vi "nanocal -- nuclear schottky fit V8.vi"() -> ()   [LabVIEW 2021] (continued)
,  \"τN\" -> 0.000008203122   ,  \"τC\" -> 0.002636418134   ,  \"κ0\" -> 0.000000022540   ,  \"mm1\" -> 0.000036639898   ,  \"mm2\" -> 0.012730445827   ,  \"mm3\" -> 0.021569578789   ,  \"T\" -> 3.100000000000   ,  \"B\" -> 10.000000000000   ,  \"θ\" -> 90.000000000000   ,  \"Reoff\" -> -204081.632653061300   ,  \"Imoff\" -> 0.000000000000   ,  \"στ1\" -> 0.714525927996   ,  \"στS\" -> 0.000197909015   ,  \"στN\" -> 0.366603423191   ,  \"τ11 \" -> 0.000000000000   ,  \"τ12\" -> 0.000000000000   ,  \"τ22\" -> 0.000000000000   ,  \"τN1\" -> 0.000000000000   ,  \"τN2\" -> 0.000000000000   ,  \"σηlogτ1 \" -> 0.000000000000   ,  \"σηlogτS\" -> 0.000000000000   ,  \"σηlogτN\" -> 0.000000000000   ,  \"σlogτ1\" -> 0.000000000000   ,  \"σlogτS\" -> 0.000000000000   ,  \"σlogτN\" -> 0.000000000000   ,  \"σητ1\" -> 0.000000000000   ,  \"σητS \" -> 0.000000000000   ,  \"σητN\" -> 0.000000000000    |>   , \n\"IDS0637_220612_RAW_cal__sam_\" ->   <|    \"ζ\" -> 0.000000000000   ,  \"τ1\" -> 0.000000000000   ,  \"τS\" -> 0.000000000000   ,  \"τN\" -> 0.000000000000   ,  \"τC\" -> 0.000000000000   ,  \"κ0\" -> 0.000000000000   ,  \"mm1\" -> 0.000000000000   ,  \"mm2\" -> 0.000000000000   ,  \"mm3\" -> 0.000000000000   ,  \"T\" -> 3.100000000000   ,  \"B\" -> 10.000000000000   ,  \"θ\" -> 90.000000000000   ,  \"Reoff\" -> 0.000000000000   ,  \"Imoff\" -> 0.000000000000   ,  \"στ1\" -> 0.000000000000   ,  \"στS\" -> 0.000000000000   ,  \"στN\" -> 0.000000000000   ,  \"τ11 \" -> 0.000000000000   ,  \"τ12\" -> 0.000000000000   ,  \"τ22\" -> 0.000000000000   ,  \"τN1\" -> 0.000000000000   ,  \"τN2\" -> 0.000000000000   ,  \"σηlogτ1 \" -> 0.000000000000   ,  \"σηlogτS\" -> 0.000000000000   ,  \"σηlogτN\" -> 0.000000000000   ,  \"σlogτ1\" -> 0.000000000000   ,  \"σlogτS\" -> 0.000000000000   ,  \"σlogτN\" -> 0.000000000000   ,  \"σητ1\" -> 0.000000000000   ,  \"σητS \" -> 0.000000000000   ,  \"σητN\" -> 0.000000000000    |>   , \n\"IDS0638_220612_RAW_cal__ref_\" ->   <|    \"ζ\" -> 0.021698598791   ,  \"τ1\" -> 0.021496688345   ,  \"τS\" -> 0.006445256992   ,  \"τN\" -> 0.000001238561   ,  \"τC\" -> 0.001823286983   ,  \"κ0\" -> 0.000000055353   ,  \"mm1\" -> 0.000030436072   ,  \"mm2\" -> 0.008377153736   ,  \"mm3\" -> 0.021498760993   ,  \"T\" -> 5.700000000000   ,  \"B\" -> 10.000000000000   ,  \"θ\" -> 90.000000000000   ,  \"Reoff\" -> -122448.979591835290   ,  \"Imoff\" -> 0.000000000000   ,  \"στ1\" -> 9.353728365028   ,  \"στS\" -> 0.000421905194   ,  \"στN\" -> 5.932285308296   ,  \"τ11 \" -> 0.000000000000   ,  \"τ12\" -> 0.000000000000   ,  \"τ22\" -> 0.000000000000   ,  \"τN1\" -> 0.000000000000   ,  \"τN2\" -> 0.000000000000   ,  \"σηlogτ1 \" -> 0.000000000000   ,  \"σηlogτS\" -> 0.000000000000   ,  \"σηlogτN\" -> 0.000000000000   ,  \"σlogτ1\" -> 0.000000000000   ,  \"σlogτS\" -> 0.000000000000   ,  \"σlogτN\" -> 0.000000000000   ,  \"σητ1\" -> 0.000000000000   ,  \"σητS \" -> 0.000000000000   ,  \"σητN\" -> 0.000000000000    |>   , \n\"IDS0638_220612_RAW_cal__sam_\" ->   <|    \"ζ\" -> 0.000000000000   ,  \"τ1\" -> 0.000000000000   ,  \"τS\" -> 0.000000000000   ,  \"τN\" -> 0.000000000000   ,  \"τC\" -> 0.000000000000   ,  \"κ0\" -> 0.000000000000   ,  \"mm1\" -> 0.000000000000   ,  \"mm2\" -> 0.000000000000   ,  \"mm3\" -> 0.000000000000   ,  \"T\" -> 5.700000000000   ,  \"B\" -> 10.000000000000   ,  \"θ\" -> 90.000000000000   ,  \"Reoff\" -> 0.000000000000   ,  \"Imoff\" -> 0.000000000000   ,  \"στ1\" -> 0.000000000000   ,  \"στS\" -> 0.000000000000   ,  \"στN\" -> 0.000000000000   ,  \"τ11 \" -> 0.000000000000   ,  \"τ12\" -> 0.000000000000   ,  \"τ22\" -> 0.000000000000   ,  \"τN1\" -> 0.000000000000   ,  \"τN2\" -> 0.000000000000   ,  \"σηlogτ1 \" -> 0.000000000000   ,  \"σηlogτS\" -> 0.000000000000   ,  \"σηlogτN\" -> 0.000000000000   ,  \"σlogτ1\" -> 0.000000000000   ,  \"σlogτS\" -> 0.000000000000   ,  \"σlogτN\" -> 0.000000000000   ,  \"σητ1\" -> 0.000000000000   ,  \"σητS \" -> 0.000000000000   ,  \"σητN\" -> 0.000000000000    |>   , \n\"IDS0640_220612_RAW_cal__ref_\" ->   <|    \"ζ\" -> 0.230099904219   ,  \"τ1\" -> 0.019803524287   ,  \"τS\" -> 0.072771074412   ,  \"τN\" -> 0.019721178899   ,  \"τC\" -> 0.000908013791   ,  \"κ0\" -> 0.000000000947   ,  \"mm1\" -> 0.000168456164   ,  \"mm2\" -> 0.014977374492   ,  \"mm3\" -> 0.119340419361   ,  \"T\" -> 0.200000000000   ,  \"B\" -> 6.000000000000   ,  \"θ\" -> 90.000000000000   ,  \"Reoff\" -> 0.000000000000   ,  \"Imoff\" -> 0.000000000000   ,  \"στ1\" -> 0.000071902729   ,  \"στS\" -> 0.000035418419   ,  \"στN\" -> 0.000036759818   ,  \"τ11 \" -> 0.000000000000   ,  \"τ12\" -> 0.000000000000   ,  \"τ22\" -> 0.000000000000   ,  \"τN1\" -> 0.000000000000   ,  \"τN2\" -> 0.000000000000   ,  \"σηlogτ1 \" -> 0.251384540647   ,  \"σηlogτS\" -> 0.006630640632   ,  \"σηlogτN\" -> 0.159565745714   ,  \"σlogτ1\" -> 0.003630804676   ,  \"σlogτS\" -> 0.000486710132   ,  \"σlogτN\" -> 0.001863976680   ,  \"σητ1\" -> 0.004978299856   ,  \"σητS \" -> 0.000482518843   ,  \"σητN\" -> 0.003146824617    |>   , \n\"IDS0640_220612_RAW_cal__sam_\" ->   <|    \"ζ\" -> 0.000000000000   ,  \"τ1\" -> 0.000000000000   ,  \"τS\" -> 0.000000000000   ,  \"τN\" -> 0.000000000000   ,  \"τC\" -> 0.000000000000   ,  \"κ0\" -> 0.000000000000   ,  \"mm1\" -> 0.000000000000   ,  \"mm2\" -> 0.000000000000   ,  \"mm3\" -> 0.000000000000   ,  \"T\" -> 0.200000000000   ,  \"B\" -> 6.000000000000   ,  \"θ\" -> 90.000000000000   ,  \"Reoff\" -> 0.000000000000   ,  \"Imoff\" -> 0.000000000000   ,  \"στ1\" -> 0.000000000000   ,  \"στS\" -> 0.000000000000   ,  \"στN\" -> 0.000000000000   ,  \"τ11 \" -> 0.000000000000   ,  \"τ12\" -> 0.000000000000   ,  \"τ22\" -> 0.000000000000   ,  \"τN1\" -> 0.000000000000   ,  \"τN2\" -> 0.000000000000   ,  \"σηlogτ1 \" -> 0.000000000000   ,  \"σηlogτS\" -> 0.000000000000   ,  \"σηlogτN\" -> 0.000000000000   ,  \"σlogτ1\" -> 0.000000000000   ,  \"σlogτS\" -> 0.000000000000   ,  \"σlogτN\" -> 0.000000000000   ,  \"σητ1\" -> 0.000000000000   ,  \"σητS \" -> 0.000000000000   ,  \"σητN\" -> 0.000000000000    |>   , \n\"IDS0641_220612_RAW_cal__ref_\" ->   <|    \"ζ\" -> 0.331411916516   ,  \"τ1\" -> 0.027436942180   ,  \"τS\" -> 0.091259190003   ,  \"τN\" -> 0.036352249292   ,  \"τC\" -> 0.000814813533   ,  \"κ0\" -> 0.000000000745   ,  \"mm1\" -> 0.000201800322   ,  \"mm2\" -> 0.018690769513   ,  \"mm3\" -> 0.179262576838   ,  \"T\" -> 0.170000000000   ,  \"B\" -> 6.000000000000   ,  \"θ\" -> 90.000000000000   ,  \"Reoff\" -> 0.000000000000   ,  \"Imoff\" -> 0.000000000000   ,  \"στ1\" -> 0.000134182156   ,  \"στS\" -> 0.000082842638   ,  \"στN\" -> 0.000089641447   ,  \"τ11 \" -> 0.000000000000   ,  \"τ12\" -> 0.000000000000   ,  \"τ22\" -> 0.000000000000   ,  \"τN1\" -> 0.000000000000   ,  \"τN2\" -> 0.000000000000   ,  \"σηlogτ1 \" -> 0.243050215213   ,  \"σηlogτS\" -> 0.008562643138   ,  \"σηlogτN\" -> 0.162803839532   ,  \"σlogτ1\" -> 0.004890565241   ,  \"σlogτS\" -> 0.000907773107   ,  \"σlogτN\" -> 0.002465911967   ,  \"σητ1\" -> 0.006668554702   ,  \"σητS \" -> 0.000781419877   ,  \"σητN\" -> 0.005918285760    |>   , \n\"IDS0641_220612_RAW_cal__sam_\" ->   <|    \"ζ\" -> 0.000000000000   ,  \"τ1\" -> 0.000000000000   ,  \"τS\" -> 0.000000000000   ,  \"τN\" -> 0.000000000000   ,  \"τC\" -> 0.000000000000   ,  \"κ0\" -> 0.000000000000   ,  \"mm1\" -> 0.000000000000   ,  \"mm2\" -> 0.000000000000   ,  \"mm3\" -> 0.000000000000   ,  \"T\" -> 0.170000000000   ,  \"B\" -> 6.000000000000   ,  \"θ\" -> 90.000000000000   ,  \"Reoff\" -> 0.000000000000   ,  \"Imoff\" -> 0.000000000000   ,  \"στ1\" -> 0.000000000000   ,  \"στS\" -> 0.000000000000   ,  \"στN\" -> 0.000000000000   ,  \"τ11 \" -> 0.000000000000   ,  \"τ12\" -> 0.000000000000   ,  \"τ22\" -> 0.000000000000   ,  \"τN1\" -> 0.000000000000   ,  \"τN2\" -> 0.000000000000   ,  \"σηlogτ1 \" -> 0.000000000000   ,  \"σηlogτS\" -> 0.000000000000   ,  \"σηlogτN\" -> 0.000000000000   ,  \"σlogτ1\" -> 0.000000000000   ,  \"σlogτS\" -> 0.000000000000   ,  \"σlogτN\" -> 0.000000000000   ,  \"σητ1\" -> 0.000000000000   ,  \"σητS \" -> 0.000000000000   ,  \"σητN\" -> 0.000000000000    |>   , \n\"IDS0642_220612_RAW_cal__ref_\" ->   <|    \"ζ\" -> 0.410773621242   ,  \"τ1\" -> 0.031455114933   ,  \"τS\" -> 0.109824084123   ,  \"τN\" -> 0.054894161716   ,  \"τC\" -> 0.000807067579   ,  \"κ0\" -> 0.000000000644   ,  \"mm1\" -> 0.000234124076   ,  \"mm2\" -> 0.020015527109   ,  \"mm3\" -> 0.244392687495   ,  \"T\" -> 0.150000000000   ,  \"B\" -> 6.000000000000   ,  \"θ\" -> 90.000000000000   ,  \"Reoff\" -> 0.000000000000   ,  \"Imoff\" -> 0.000000000000   ,  \"στ1\" -> 0.000244365389   ,  \"στS\" -> 0.000194798011   ,  \"στN\" -> 0.000213345438   ,  \"τ11 \" -> 0.000000000000   ,  \"τ12\" -> 0.000000000000   ,  \"τ22\" -> 0.000000000000   ,  \"τN1\" -> 0.000000000000   ,  \"τN2\" -> 0.000000000000   ,  \"σηlogτ1 \" -> 0.251218681926   ,  \"σηlogτS\" -> 0.010865743955   ,  \"σηlogτN\" -> 0.168296468755   ,  \"σlogτ1\" -> 0.007768701196   ,  \"σlogτS\" -> 0.001773727614   ,  \"σlogτN\" -> 0.003886486855   ,  \"σητ1\" -> 0.007902112513   ,  \"σητS \" -> 0.001193320378   ,  \"σητN\" -> 0.009238493572    |>   , \n\"IDS0642_220612_RAW_cal__sam_\" ->   <|    \"ζ\" -> 0.000000000000   ,  \"τ1\" -> 0.000000000000   ,  \"τS\" -> 0.000000000000   ,  \"τN\" -> 0.000000000000   ,  \"τC\" -> 0.000000000000   ,  \"κ0\" -> 0.000000000000   ,  \"mm1\" -> 0.000000000000   ,  \"mm2\" -> 0.000000000000   ,  \"mm3\" -> 0.000000000000   ,  \"T\" -> 0.150000000000   ,  \"B\" -> 6.000000000000   ,  \"θ\" -> 90.000000000000   ,  \"Reoff\" -> 0.000000000000   ,  \"Imoff\" -> 0.000000000000   ,  \"στ1\" -> 0.000000000000   ,  \"στS\" -> 0.000000000000   ,  \"στN\" -> 0.000000000000   ,  \"τ11 \" -> 0.000000000000   ,  \"τ12\" -> 0.000000000000   ,  \"τ22\" -> 0.000000000000   ,  \"τN1\" -> 0.000000000000   ,  \"τN2\" -> 0.000000000000   ,  \"σηlogτ1 \" -> 0.000000000000   ,  \"σηlogτS\" -> 0.000000000000   ,  \"σηlogτN\" -> 0.000000000000   ,  \"σlogτ1\" -> 0.000000000000   ,  \"σlogτS\" -> 0.000000000000   ,  \"σlogτN\" -> 0.000000000000   ,  \"σητ1\" -> 0.000000000000   ,  \"σητS \" -> 0.000000000000   ,  \"σητN\" -> 0.000000000000    |>   , \n\"IDS0643_220612_RAW_cal__ref_\" ->   <|    \"ζ\" -> 0.645665826507   ,  \"τ1\" -> 0.033591555956   ,  \"τS\" -> 0.115598019979   ,  \"τN\" -> 0.189817561833   ,  \"τC\" -> 0.000794602780   ,  \"κ0\" -> 0.000000000472   ,  \"mm1\" -> 0.000310954135   ,  \"mm2\" -> 0.012215752320   ,  \"mm3\" -> 0.524471438152   ,  \"T\" -> 0.120000000000   ,  \"B\" -> 6.000000000000   ,  \"θ\" -> 90.000000000000   ,  \"Reoff\" -> -174187755.102040827000   ,  \"Imoff\" -> 0.000000000000   ,  \"στ1\" -> 0.039640874529   ,  \"στS\" -> 0.065981071320   ,  \"στN\" -> 0.095740947662   ,  \"τ11 \" -> 0.000000000000   ,  \"τ12\" -> 0.000000000000   ,  \"τ22\" -> 0.000000000000   ,  \"τN1\" -> 0.000000000000   ,  \"τN2\" -> 0.000000000000   ,  \"σηlogτ1 \" -> 0.000000000000   ,  \"σηlogτS\" -> 0.000000000000   ,  \"σηlogτN\" -> 0.000000000000   ,  \"σlogτ1\" -> 0.000000000000   ,  \"σlogτS\" -> 0.000000000000   ,  \"σlogτN\" -> 0.000000000000   ,  \"σητ1\" -> 0.000000000000   ,  \"σητS \" -> 0.000000000000   ,  \"σητN\" -> 0.000000000000    |>   , \n\"IDS0643_220612_RAW_cal__sam_\" ->   <|    \"ζ\" -> 0.000000000000   ,  \"τ1\" -> 0.000000000000   ,  \"τS\" -> 0.000000000000   ,  \"τN\" -> 0.000000000000   ,  \"τC\" -> 0.000000000000   ,  \"κ0\" -> 0.000000000000   ,  \"mm1\" -> 0.000000000000   ,  \"mm2\" -> 0.000000000000   ,  \"mm3\" -> 0.000000000000   ,  \"T\" -> 0.120000000000   ,  \"B\" -> 6.000000000000   ,  \"θ\" -> 90.000000000000   ,  \"Reoff\" -> 0.000000000000   ,  \"Imoff\" -> 0.000000000000   ,  \"στ1\" -> 0.000000000000   ,  \"στS\" -> 0.000000000000   ,  \"στN\" -> 0.000000000000   ,  \"τ11 \" -> 0.000000000000   ,  \"τ12\" -> 0.000000000000   ,  \"τ22\" -> 0.000000000000   ,  \"τN1\" -> 0.000000000000   ,  \"τN2\" -> 0.000000000000   ,  \"σηlogτ1 \" -> 0.000000000000   ,  \"σηlogτS\" -> 0.000000000000   ,  \"σηlogτN\" -> 0.000000000000   ,  \"σlogτ1\" -> 0.000000000000   ,  \"σlogτS\" -> 0.000000000000   ,  \"σlogτN\" -> 0.000000000000   ,  \"σητ1\" -> 0.000000000000   ,  \"σητS \" -> 0.000000000000   ,  \"σητN\" -> 0.000000000000    |>   , \n\"IDS0644_220612_RAW_cal__ref_\" ->   <|    \"ζ\" -> 0.157159831769   ,  \"τ1\" -> 0.017275661419   ,  \"τS\" -> 0.057507819747   ,  \"τN\" -> 0.009018768853   ,  \"τC\" -> 0.000968005523   ,  \"κ0\" -> 0.000000001253   ,  \"mm1\" -> 0.000129832569   ,  \"mm2\" -> 0.014431696620   ,  \"mm3\" -> 0.080664033825   ,  \"T\" -> 0.250000000000   ,  \"B\" -> 6.000000000000   ,  \"θ\" -> 90.000000000000   ,  \"Reoff\" -> 0.000000000000   ,  \"Imoff\" -> 0.000000000000   ,  \"στ1\" -> 0.000090637790   ,  \"στS\" -> 0.000023650584   ,  \"στN\" -> 0.000024208134   ,  \"τ11 \" -> 0.000000000000   ,  \"τ12\" -> 0.000000000000   ,  \"τ22\" -> 0.000000000000   ,  \"τN1\" -> 0.000000000000   ,  \"τN2\" -> 0.000000000000   ,  \"σηlogτ1 \" -> 0.236297448492   ,  \"σηlogτS\" -> 0.003600470511   ,  \"σηlogτN\" -> 0.153004528887   ,  \"σlogτ1\" -> 0.005246559741   ,  \"σlogτS\" -> 0.000411258583   ,  \"σlogτN\" -> 0.002684194999   ,  \"σητ1\" -> 0.004082194714   ,  \"σητS \" -> 0.000207055209   ,  \"σητN\" -> 0.001379912479    |>   , \n\"IDS0644_220612_RAW_cal__sam_\" ->   <|    \"ζ\" -> 0.000000000000   ,  \"τ1\" -> 0.000000000000   ,  \"τS\" -> 0.000000000000   ,  \"τN\" -> 0.000000000000   ,  \"τC\" -> 0.000000000000   ,  \"κ0\" -> 0.000000000000   ,  \"mm1\" -> 0.000000000000   ,  \"mm2\" -> 0.000000000000   ,  \"mm3\" -> 0.000000000000   ,  \"T\" -> 0.250000000000   ,  \"B\" -> 6.000000000000   ,  \"θ\" -> 90.000000000000   ,  \"Reoff\" -> 0.000000000000   ,  \"Imoff\" -> 0.000000000000   ,  \"στ1\" -> 0.000000000000   ,  \"στS\" -> 0.000000000000   ,  \"στN\" -> 0.000000000000   ,  \"τ11 \" -> 0.000000000000   ,  \"τ12\" -> 0.000000000000   ,  \"τ22\" -> 0.000000000000   ,  \"τN1\" -> 0.000000000000   ,  \"τN2\" -> 0.000000000000   ,  \"σηlogτ1 \" -> 0.000000000000   ,  \"σηlogτS\" -> 0.000000000000   ,  \"σηlogτN\" -> 0.000000000000   ,  \"σlogτ1\" -> 0.000000000000   ,  \"σlogτS\" -> 0.000000000000   ,  \"σlogτN\" -> 0.000000000000   ,  \"σητ1\" -> 0.000000000000   ,  \"σητS \" -> 0.000000000000   ,  \"σητN\" -> 0.000000000000    |>   , \n\"IDS0645_220612_RAW_cal__ref_\" ->   <|    \"ζ\" -> 0.108151444543   ,  \"τ1\" -> 0.016704569544   ,  \"τS\" -> 0.049250197086   ,  \"τN\" -> 0.004328811909   ,  \"τC\" -> 0.001175701627   ,  \"κ0\" -> 0.000000001596   ,  \"mm1\" -> 0.000112550307   ,  \"mm2\" -> 0.014943415376   ,  \"mm3\" -> 0.062197961702   ,  \"T\" -> 0.300000000000   ,  \"B\" -> 6.000000000000   ,  \"θ\" -> 90.000000000000   ,  \"Reoff\" -> 0.000000000000   ,  \"Imoff\" -> 0.000000000000   ,  \"στ1\" -> 0.000153951281   ,  \"στS\" -> 0.000019651803   ,  \"στN\" -> 0.000020146314   ,  \"τ11 \" -> 0.000000000000   ,  \"τ12\" -> 0.000000000000   ,  \"τ22\" -> 0.000000000000   ,  \"τN1\" -> 0.000000000000   ,  \"τN2\" -> 0.000000000000   ,  \"σηlogτ1 \" -> 0.218575565601   ,  \"σηlogτS\" -> 0.001786286514   ,  \"σηlogτN\" -> 0.148268126955   ,  \"σlogτ1\" -> 0.009216117846   ,  \"σlogτS\" -> 0.000399019782   ,  \"σlogτN\" -> 0.004654005435   ,  \"σητ1\" -> 0.003651210736   ,  \"σητS \" -> 0.000087974963   ,  \"σητN\" -> 0.000641824834    |>   , \n\"IDS0645_220612_RAW_cal__sam_\" ->   <|    \"ζ\" -> 0.000000000000   ,  \"τ1\" -> 0.000000000000   ,  \"τS\" -> 0.000000000000   ,  \"τN\" -> 0.000000000000   ,  \"τC\" -> 0.000000000000   ,  \"κ0\" -> 0.000000000000   ,  \"mm1\" -> 0.000000000000   ,  \"mm2\" -> 0.000000000000   ,  \"mm3\" -> 0.000000000000   ,  \"T\" -> 0.300000000000   ,  \"B\" -> 6.000000000000   ,  \"θ\" -> 90.000000000000   ,  \"Reoff\" -> 0.000000000000   ,  \"Imoff\" -> 0.000000000000   ,  \"στ1\" -> 0.000000000000   ,  \"στS\" -> 0.000000000000   ,  \"στN\" -> 0.000000000000   ,  \"τ11 \" -> 0.000000000000   ,  \"τ12\" -> 0.000000000000   ,  \"τ22\" -> 0.000000000000   ,  \"τN1\" -> 0.000000000000   ,  \"τN2\" -> 0.000000000000   ,  \"σηlogτ1 \" -> 0.000000000000   ,  \"σηlogτS\" -> 0.000000000000   ,  \"σηlogτN\" -> 0.000000000000   ,  \"σlogτ1\" -> 0.000000000000   ,  \"σlogτS\" -> 0.000000000000   ,  \"σlogτN\" -> 0.000000000000   ,  \"σητ1\" -> 0.000000000000   ,  \"σητS \" -> 0.000000000000   ,  \"σητN\" -> 0.000000000000    |>   , \n\"IDS0646_220612_RAW_cal__ref_\" ->   <|    \"ζ\" -> 0.077732977787   ,  \"τ1\" -> 0.018222452777   ,  \"τS\" -> 0.042664974364   ,  \"τN\" -> 0.002414957753   ,  \"τC\" -> 0.001447490324   ,  \"κ0\" -> 0.000000001997   ,  \"mm1\" -> 0.000101431981   ,  \"mm2\" -> 0.016791513450   ,  \"mm3\" -> 0.051361127148   ,  \"T\" -> 0.360000000000   ,  \"B\" -> 6.000000000000   ,  \"θ\" -> 90.000000000000   ,  \"Reoff\" -> 0.000000000000   ,  \"Imoff\" -> 0.000000000000   ,  \"στ1\" -> 0.000164595012   ,  \"στS\" -> 0.000010037791   ,  \"στN\" -> 0.000010800479   ,  \"τ11 \" -> 0.000000000000   ,  \"τ12\" -> 0.000000000000   ,  \"τ22\" -> 0.000000000000   ,  \"τN1\" -> 0.000000000000   ,  \"τN2\" -> 0.000000000000   ,  \"σηlogτ1 \" -> 0.189495281548   ,  \"σηlogτS\" -> 0.000864174070   ,  \"σηlogτN\" -> 0.143351503659   ,  \"σlogτ1\" -> 0.009032538816   ,  \"σlogτS\" -> 0.000235270067   ,  \"σlogτN\" -> 0.004472326314   ,  \"σητ1\" -> 0.003453068820   ,  \"σητS \" -> 0.000036869965   ,  \"σητN\" -> 0.000346187825    |>   , \n\"IDS0646_220612_RAW_cal__sam_\" ->   <|    \"ζ\" -> 0.000000000000   ,  \"τ1\" -> 0.000000000000   ,  \"τS\" -> 0.000000000000   ,  \"τN\" -> 0.000000000000   ,  \"τC\" -> 0.000000000000   ,  \"κ0\" -> 0.000000000000   ,  \"mm1\" -> 0.000000000000   ,  \"mm2\" -> 0.000000000000   ,  \"mm3\" -> 0.000000000000   ,  \"T\" -> 0.360000000000   ,  \"B\" -> 6.000000000000   ,  \"θ\" -> 90.000000000000   ,  \"Reoff\" -> 0.000000000000   ,  \"Imoff\" -> 0.000000000000   ,  \"στ1\" -> 0.000000000000   ,  \"στS\" -> 0.000000000000   ,  \"στN\" -> 0.000000000000   ,  \"τ11 \" -> 0.000000000000   ,  \"τ12\" -> 0.000000000000   ,  \"τ22\" -> 0.000000000000   ,  \"τN1\" -> 0.000000000000   ,  \"τN2\" -> 0.000000000000   ,  \"σηlogτ1 \" -> 0.000000000000   ,  \"σηlogτS\" -> 0.000000000000   ,  \"σηlogτN\" -> 0.000000000000   ,  \"σlogτ1\" -> 0.000000000000   ,  \"σlogτS\" -> 0.000000000000   ,  \"σlogτN\" -> 0.000000000000   ,  \"σητ1\" -> 0.000000000000   ,  \"σητS \" -> 0.000000000000   ,  \"σητN\" -> 0.000000000000    |>   , \n\"IDS0647_220612_RAW_cal__ref_\" ->   <|    \"ζ\" -> 0.059413527113   ,  \"τ1\" -> 0.016818995328   ,  \"τS\" -> 0.037585637610   ,  \"τN\" -> 0.001580842075   ,  \"τC\" -> 0.001700025734   ,  \"κ0\" -> 0.000000002392   ,  \"mm1\" -> 0.000091637686   ,  \"mm2\" -> 0.015787959466   ,  \"mm3\" -> 0.044132922297   ,  \"T\" -> 0.420000000000   ,  \"B\" -> 6.000000000000   ,  \"θ\" -> 90.000000000000   ,  \"Reoff\" -> 0.000000000000   ,  \"Imoff\" -> 0.000000000000   ,  \"στ1\" -> 0.000108112505   ,  \"στS\" -> 0.000004614270   ,  \"στN\" -> 0.000005017637   ,  \"τ11 \" -> 0.000000000000   ,  \"τ12\" -> 0.000000000000   ,  \"τ22\" -> 0.000000000000   ,  \"τN1\" -> 0.000000000000   ,  \"τN2\" -> 0.000000000000   ,  \"σηlogτ1 \" -> 0.183880264698   ,  \"σηlogτS\" -> 0.000605017197   ,  \"σηlogτN\" -> 0.142205307504   ,  \"σlogτ1\" -> 0.006428000169   ,  \"σlogτS\" -> 0.000122766832   ,  \"σlogτN\" -> 0.003174028004   ,  \"σητ1\" -> 0.003092681313   ,  \"σητS \" -> 0.000022739957   ,  \"σητN\" -> 0.000224804133    |>   , \n\"IDS0647_220612_RAW_cal__sam_\" ->   <|    \"ζ\" -> 0.000000000000   ,  \"τ1\" -> 0.000000000000   ,  \"τS\" -> 0.000000000000   ,  \"τN\" -> 0.000000000000   ,  \"τC\" -> 0.000000000000   ,  \"κ0\" -> 0.000000000000   ,  \"mm1\" -> 0.000000000000   ,  \"mm2\" -> 0.000000000000   ,  \"mm3\" -> 0.000000000000   ,  \"T\" -> 0.420000000000   ,  \"B\" -> 6.000000000000   ,  \"θ\" -> 90.000000000000   ,  \"Reoff\" -> 0.000000000000   ,  \"Imoff\" -> 0.000000000000   ,  \"στ1\" -> 0.000000000000   ,  \"στS\" -> 0.000000000000   ,  \"στN\" -> 0.000000000000   ,  \"τ11 \" -> 0.000000000000   ,  \"τ12\" -> 0.000000000000   ,  \"τ22\" -> 0.000000000000   ,  \"τN1\" -> 0.000000000000   ,  \"τN2\" -> 0.000000000000   ,  \"σηlogτ1 \" -> 0.000000000000   ,  \"σηlogτS\" -> 0.000000000000   ,  \"σηlogτN\" -> 0.000000000000   ,  \"σlogτ1\" -> 0.000000000000   ,  \"σlogτS\" -> 0.000000000000   ,  \"σlogτN\" -> 0.000000000000   ,  \"σητ1\" -> 0.000000000000   ,  \"σητS \" -> 0.000000000000   ,  \"σητN\" -> 0.000000000000    |>   , \n\"IDS0648_220613_RAW_cal__ref_\" ->   <|    \"ζ\" -> 0.044166566928   ,  \"τ1\" -> 0.016574003526   ,  \"τS\" -> 0.032211448360   ,  \"τN\" -> 0.000936709307   ,  \"τC\" -> 0.001862438862   ,  \"κ0\" -> 0.000000003065   ,  \"mm1\" -> 0.000074801958   ,  \"mm2\" -> 0.015787727605   ,  \"mm3\" -> 0.037186110816   ,  \"T\" -> 0.520000000000   ,  \"B\" -> 6.000000000000   ,  \"θ\" -> 90.000000000000   ,  \"Reoff\" -> 0.000000000000   ,  \"Imoff\" -> 0.000000000000   ,  \"στ1\" -> 0.000113368552   ,  \"στS\" -> 0.000002764404   ,  \"στN\" -> 0.000003162403   ,  \"τ11 \" -> 0.000000000000   ,  \"τ12\" -> 0.000000000000   ,  \"τ22\" -> 0.000000000000   ,  \"τN1\" -> 0.000000000000   ,  \"τN2\" -> 0.000000000000   ,  \"σηlogτ1 \" -> 0.169044191232   ,  \"σηlogτS\" -> 0.000346748172   ,  \"σηlogτN\" -> 0.139725969375   ,  \"σlogτ1\" -> 0.006840142890   ,  \"σlogτS\" -> 0.000085820552   ,  \"σlogτN\" -> 0.003376077471   ,  \"σητ1\" -> 0.002801739022   ,  \"σητS \" -> 0.000011169261   ,  \"σητN\" -> 0.000130882616    |>   , \n\"IDS0648_220613_RAW_cal__sam_\" ->   <|    \"ζ\" -> 0.000000000000   ,  \"τ1\" -> 0.000000000000   ,  \"τS\" -> 0.000000000000   ,  \"τN\" -> 0.000000000000   ,  \"τC\" -> 0.000000000000   ,  \"κ0\" -> 0.000000000000   ,  \"mm1\" -> 0.000000000000   ,  \"mm2\" -> 0.000000000000   ,  \"mm3\" -> 0.000000000000   ,  \"T\" -> 0.520000000000   ,  \"B\" -> 6.000000000000   ,  \"θ\" -> 90.000000000000   ,  \"Reoff\" -> 0.000000000000   ,  \"Imoff\" -> 0.000000000000   ,  \"στ1\" -> 0.000000000000   ,  \"στS\" -> 0.000000000000   ,  \"στN\" -> 0.000000000000   ,  \"τ11 \" -> 0.000000000000   ,  \"τ12\" -> 0.000000000000   ,  \"τ22\" -> 0.000000000000   ,  \"τN1\" -> 0.000000000000   ,  \"τN2\" -> 0.000000000000   ,  \"σηlogτ1 \" -> 0.000000000000   ,  \"σηlogτS\" -> 0.000000000000   ,  \"σηlogτN\" -> 0.000000000000   ,  \"σlogτ1\" -> 0.000000000000   ,  \"σlogτS\" -> 0.000000000000   ,  \"σlogτN\" -> 0.000000000000   ,  \"σητ1\" -> 0.000000000000   ,  \"σητS \" -> 0.000000000000   ,  \"σητN\" -> 0.000000000000    |>   , \n\"IDS0649_220613_RAW_cal__ref_\" ->   <|    \"ζ\" -> 0.036098260006   ,  \"τ1\" -> 0.019839922246   ,  \"τS\" -> 0.028557133674   ,  \"τN\" -> 0.000530751010   ,  \"τC\" -> 0.002125743780   ,  \"κ0\" -> 0.000000003752   ,  \"mm1\" -> 0.000069248734   ,  \"mm2\" -> 0.019012462838   ,  \"mm3\" -> 0.033021861162   ,  \"T\" -> 0.620000000000   ,  \"B\" -> 6.000000000000   ,  \"θ\" -> 90.000000000000   ,  \"Reoff\" -> 0.000000000000   ,  \"Imoff\" -> 0.000000000000   ,  \"στ1\" -> 0.000292189890   ,  \"στS\" -> 0.000002960548   ,  \"στN\" -> 0.000003977957   ,  \"τ11 \" -> 0.000000000000   ,  \"τ12\" -> 0.000000000000   ,  \"τ22\" -> 0.000000000000   ,  \"τN1\" -> 0.000000000000   ,  \"τN2\" -> 0.000000000000   ,  \"σηlogτ1 \" -> 0.142367105799   ,  \"σηlogτS\" -> 0.000145255254   ,  \"σηlogτN\" -> 0.135095367098   ,  \"σlogτ1\" -> 0.014727370701   ,  \"σlogτS\" -> 0.000103671054   ,  \"σlogτN\" -> 0.007494959556   ,  \"σητ1\" -> 0.002824552309   ,  \"σητS \" -> 0.000004148074   ,  \"σητN\" -> 0.000071702003    |>   , \n\"IDS0649_220613_RAW_cal__sam_\" ->   <|    \"ζ\" -> 0.000000000000   ,  \"τ1\" -> 0.000000000000   ,  \"τS\" -> 0.000000000000   ,  \"τN\" -> 0.000000000000   ,  \"τC\" -> 0.000000000000   ,  \"κ0\" -> 0.000000000000   ,  \"mm1\" -> 0.000000000000   ,  \"mm2\" -> 0.000000000000   ,  \"mm3\" -> 0.000000000000   ,  \"T\" -> 0.620000000000   ,  \"B\" -> 6.000000000000   ,  \"θ\" -> 90.000000000000   ,  \"Reoff\" -> 0.000000000000   ,  \"Imoff\" -> 0.000000000000   ,  \"στ1\" -> 0.000000000000   ,  \"στS\" -> 0.000000000000   ,  \"στN\" -> 0.000000000000   ,  \"τ11 \" -> 0.000000000000   ,  \"τ12\" -> 0.000000000000   ,  \"τ22\" -> 0.000000000000   ,  \"τN1\" -> 0.000000000000   ,  \"τN2\" -> 0.000000000000   ,  \"σηlogτ1 \" -> 0.000000000000   ,  \"σηlogτS\" -> 0.000000000000   ,  \"σηlogτN\" -> 0.000000000000   ,  \"σlogτ1\" -> 0.000000000000   ,  \"σlogτS\" -> 0.000000000000   ,  \"σlogτN\" -> 0.000000000000   ,  \"σητ1\" -> 0.000000000000   ,  \"σητS \" -> 0.000000000000   ,  \"σητN\" -> 0.000000000000    |>   , \n\"IDS0650_220613_RAW_cal__ref_\" ->   <|    \"ζ\" -> 0.026767413186   ,  \"τ1\" -> 0.019958900137   ,  \"τS\" -> 0.023153953288   ,  \"τN\" -> 0.000189088054   ,  \"τC\" -> 0.002398350564   ,  \"κ0\" -> 0.000000005121   ,  \"mm1\" -> 0.000056918136   ,  \"mm2\" -> 0.019398352629   ,  \"mm3\" -> 0.026869854112   ,  \"T\" -> 0.820000000000   ,  \"B\" -> 6.000000000000   ,  \"θ\" -> 90.000000000000   ,  \"Reoff\" -> 0.000000000000   ,  \"Imoff\" -> 0.000000000000   ,  \"στ1\" -> 0.000637008577   ,  \"στS\" -> 0.000002061875   ,  \"στN\" -> 0.000003206406   ,  \"τ11 \" -> 0.000000000000   ,  \"τ12\" -> 0.000000000000   ,  \"τ22\" -> 0.000000000000   ,  \"τN1\" -> 0.000000000000   ,  \"τN2\" -> 0.000000000000   ,  \"σηlogτ1 \" -> 0.127380236705   ,  \"σηlogτS\" -> 0.000047088453   ,  \"σηlogτN\" -> 0.132172067620   ,  \"σlogτ1\" -> 0.031916016057   ,  \"σlogτS\" -> 0.000089050669   ,  \"σlogτN\" -> 0.016957208977   ,  \"σητ1\" -> 0.002542369424   ,  \"σητS \" -> 0.000001090284   ,  \"σητN\" -> 0.000024992159    |>   , \n\"IDS0650_220613_RAW_cal__sam_\" ->   <|    \"ζ\" -> 0.000000000000   ,  \"τ1\" -> 0.000000000000   ,  \"τS\" -> 0.000000000000   ,  \"τN\" -> 0.000000000000   ,  \"τC\" -> 0.000000000000   ,  \"κ0\" -> 0.000000000000   ,  \"mm1\" -> 0.000000000000   ,  \"mm2\" -> 0.000000000000   ,  \"mm3\" -> 0.000000000000   ,  \"T\" -> 0.820000000000   ,  \"B\" -> 6.000000000000   ,  \"θ\" -> 90.000000000000   ,  \"Reoff\" -> 0.000000000000   ,  \"Imoff\" -> 0.000000000000   ,  \"στ1\" -> 0.000000000000   ,  \"στS\" -> 0.000000000000   ,  \"στN\" -> 0.000000000000   ,  \"τ11 \" -> 0.000000000000   ,  \"τ12\" -> 0.000000000000   ,  \"τ22\" -> 0.000000000000   ,  \"τN1\" -> 0.000000000000   ,  \"τN2\" -> 0.000000000000   ,  \"σηlogτ1 \" -> 0.000000000000   ,  \"σηlogτS\" -> 0.000000000000   ,  \"σηlogτN\" -> 0.000000000000   ,  \"σlogτ1\" -> 0.000000000000   ,  \"σlogτS\" -> 0.000000000000   ,  \"σlogτN\" -> 0.000000000000   ,  \"σητ1\" -> 0.000000000000   ,  \"σητS \" -> 0.000000000000   ,  \"σητN\" -> 0.000000000000    |>   , \n\"IDS0651_220613_RAW_cal__ref_\" ->   <|    \"ζ\" -> 0.024620092111   ,  \"τ1\" -> 0.015537036119   ,  \"τS\" -> 0.019312906027   ,  \"τN\" -> 0.000067030104   ,  \"τC\" -> 0.002705916622   ,  \"κ0\" -> 0.000000007154   ,  \"mm1\" -> 0.000057343864   ,  \"mm2\" -> 0.015387205435   ,  \"mm3\" -> 0.022655475386   ,  \"T\" -> 1.120000000000   ,  \"B\" -> 6.000000000000   ,  \"θ\" -> 90.000000000000   ,  \"Reoff\" -> 0.000000000000   ,  \"Imoff\" -> 0.000000000000   ,  \"στ1\" -> 0.001880910040   ,  \"στS\" -> 0.000002935864   ,  \"στN\" -> 0.000004201788   ,  \"τ11 \" -> 0.000000000000   ,  \"τ12\" -> 0.000000000000   ,  \"τ22\" -> 0.000000000000   ,  \"τN1\" -> 0.000000000000   ,  \"τN2\" -> 0.000000000000   ,  \"σηlogτ1 \" -> 0.134633854477   ,  \"σηlogτS\" -> 0.000023496461   ,  \"σηlogτN\" -> 0.133516099454   ,  \"σlogτ1\" -> 0.121059771335   ,  \"σlogτS\" -> 0.000152015645   ,  \"σlogτN\" -> 0.062685083512   ,  \"σητ1\" -> 0.002091811060   ,  \"σητS \" -> 0.000000453785   ,  \"σητN\" -> 0.000008949598    |>   , \n\"IDS0651_220613_RAW_cal__sam_\" ->   <|    \"ζ\" -> 0.000000000000   ,  \"τ1\" -> 0.000000000000   ,  \"τS\" -> 0.000000000000   ,  \"τN\" -> 0.000000000000   ,  \"τC\" -> 0.000000000000   ,  \"κ0\" -> 0.000000000000   ,  \"mm1\" -> 0.000000000000   ,  \"mm2\" -> 0.000000000000   ,  \"mm3\" -> 0.000000000000   ,  \"T\" -> 1.120000000000   ,  \"B\" -> 6.000000000000   ,  \"θ\" -> 90.000000000000   ,  \"Reoff\" -> 0.000000000000   ,  \"Imoff\" -> 0.000000000000   ,  \"στ1\" -> 0.000000000000   ,  \"στS\" -> 0.000000000000   ,  \"στN\" -> 0.000000000000   ,  \"τ11 \" -> 0.000000000000   ,  \"τ12\" -> 0.000000000000   ,  \"τ22\" -> 0.000000000000   ,  \"τN1\" -> 0.000000000000   ,  \"τN2\" -> 0.000000000000   ,  \"σηlogτ1 \" -> 0.000000000000   ,  \"σηlogτS\" -> 0.000000000000   ,  \"σηlogτN\" -> 0.000000000000   ,  \"σlogτ1\" -> 0.000000000000   ,  \"σlogτS\" -> 0.000000000000   ,  \"σlogτN\" -> 0.000000000000   ,  \"σητ1\" -> 0.000000000000   ,  \"σητS \" -> 0.000000000000   ,  \"σητN\" -> 0.000000000000    |>   , \n\"IDS0652_220613_RAW_cal__ref_\" ->   <|    \"ζ\" -> 0.018133168210   ,  \"τ1\" -> 0.015564889407   ,  \"τS\" -> 0.014281099211   ,  \"τN\" -> 0.000013869214   ,  \"τC\" -> 0.003052925154   ,  \"κ0\" -> 0.000000012545   ,  \"mm1\" -> 0.000045053166   ,  \"mm2\" -> 0.015460375194   ,  \"mm3\" -> 0.017666567693   ,  \"T\" -> 1.900000000000   ,  \"B\" -> 6.000000000000   ,  \"θ\" -> 90.000000000000   ,  \"Reoff\" -> 0.000000000000   ,  \"Imoff\" -> 0.000000000000   ,  \"στ1\" -> 0.007531531497   ,  \"στS\" -> 0.000002103829   ,  \"στN\" -> 0.000003717358   ,  \"τ11 \" -> 0.000000000000   ,  \"τ12\" -> 0.000000000000   ,  \"τ22\" -> 0.000000000000   ,  \"τN1\" -> 0.000000000000   ,  \"τN2\" -> 0.000000000000   ,  \"σηlogτ1 \" -> 0.117619771927   ,  \"σηlogτS\" -> 0.000004424081   ,  \"σηlogτN\" -> 0.130136475948   ,  \"σlogτ1\" -> 0.483879538125   ,  \"σlogτS\" -> 0.000147315653   ,  \"σlogτN\" -> 0.268029442413   ,  \"σητ1\" -> 0.001830738742   ,  \"σητS \" -> 0.000000063181   ,  \"σητN\" -> 0.000001804891    |>   , \n\"IDS0652_220613_RAW_cal__sam_\" ->   <|    \"ζ\" -> 0.000000000000   ,  \"τ1\" -> 0.000000000000   ,  \"τS\" -> 0.000000000000   ,  \"τN\" -> 0.000000000000   ,  \"τC\" -> 0.000000000000   ,  \"κ0\" -> 0.000000000000   ,  \"mm1\" -> 0.000000000000   ,  \"mm2\" -> 0.000000000000   ,  \"mm3\" -> 0.000000000000   ,  \"T\" -> 1.900000000000   ,  \"B\" -> 6.000000000000   ,  \"θ\" -> 90.000000000000   ,  \"Reoff\" -> 0.000000000000   ,  \"Imoff\" -> 0.000000000000   ,  \"στ1\" -> 0.000000000000   ,  \"στS\" -> 0.000000000000   ,  \"στN\" -> 0.000000000000   ,  \"τ11 \" -> 0.000000000000   ,  \"τ12\" -> 0.000000000000   ,  \"τ22\" -> 0.000000000000   ,  \"τN1\" -> 0.000000000000   ,  \"τN2\" -> 0.000000000000   ,  \"σηlogτ1 \" -> 0.000000000000   ,  \"σηlogτS\" -> 0.000000000000   ,  \"σηlogτN\" -> 0.000000000000   ,  \"σlogτ1\" -> 0.000000000000   ,  \"σlogτS\" -> 0.000000000000   ,  \"σlogτN\" -> 0.000000000000   ,  \"σητ1\" -> 0.000000000000   ,  \"σητS \" -> 0.000000000000   ,  \"σητN\" -> 0.000000000000    |>   , \n\"IDS0653_220613_RAW_cal__ref_\" ->   <|    \"ζ\" -> 0.015908509188   ,  \"τ1\" -> 0.015560123784   ,  \"τS\" -> 0.010437245612   ,  \"τN\" -> 0.000002583564   ,  \"τC\" -> 0.002705916622   ,  \"κ0\" -> 0.000000022391   ,  \"mm1\" -> 0.000033844139   ,  \"mm2\" -> 0.013260236097   ,  \"mm3\" -> 0.015577871465   ,  \"T\" -> 3.100000000000   ,  \"B\" -> 6.000000000000   ,  \"θ\" -> 90.000000000000   ,  \"Reoff\" -> 0.000000000000   ,  \"Imoff\" -> 0.000000000000   ,  \"στ1\" -> 0.028222346539   ,  \"στS\" -> 0.000001217229   ,  \"στN\" -> 0.000002849695   ,  \"τ11 \" -> 0.000000000000   ,  \"τ12\" -> 0.000000000000   ,  \"τ22\" -> 0.000000000000   ,  \"τN1\" -> 0.000000000000   ,  \"τN2\" -> 0.000000000000   ,  \"σηlogτ1 \" -> 0.102372166935   ,  \"σηlogτS\" -> 0.000000706034   ,  \"σηlogτN\" -> 0.126762129997   ,  \"σlogτ1\" -> 1.813761055527   ,  \"σlogτS\" -> 0.000116623590   ,  \"σlogτN\" -> 1.103009360706   ,  \"σητ1\" -> 0.001592923590   ,  \"σητS \" -> 0.000000007369   ,  \"σητN\" -> 0.000000327498    |>   , \n\"IDS0653_220613_RAW_cal__sam_\" ->   <|    \"ζ\" -> 0.000000000000   ,  \"τ1\" -> 0.000000000000   ,  \"τS\" -> 0.000000000000   ,  \"τN\" -> 0.000000000000   ,  \"τC\" -> 0.000000000000   ,  \"κ0\" -> 0.000000000000   ,  \"mm1\" -> 0.000000000000   ,  \"mm2\" -> 0.000000000000   ,  \"mm3\" -> 0.000000000000   ,  \"T\" -> 3.100000000000   ,  \"B\" -> 6.000000000000   ,  \"θ\" -> 90.000000000000   ,  \"Reoff\" -> 0.000000000000   ,  \"Imoff\" -> 0.000000000000   ,  \"στ1\" -> 0.000000000000   ,  \"στS\" -> 0.000000000000   ,  \"στN\" -> 0.000000000000   ,  \"τ11 \" -> 0.000000000000   ,  \"τ12\" -> 0.000000000000   ,  \"τ22\" -> 0.000000000000   ,  \"τN1\" -> 0.000000000000   ,  \"τN2\" -> 0.000000000000   ,  \"σηlogτ1 \" -> 0.000000000000   ,  \"σηlogτS\" -> 0.000000000000   ,  \"σηlogτN\" -> 0.000000000000   ,  \"σlogτ1\" -> 0.000000000000   ,  \"σlogτS\" -> 0.000000000000   ,  \"σlogτN\" -> 0.000000000000   ,  \"σητ1\" -> 0.000000000000   ,  \"σητS \" -> 0.000000000000   ,  \"σητN\" -> 0.000000000000    |>   , \n\"IDS0654_220613_RAW_cal__ref_\" ->   <|    \"ζ\" -> 0.019038104176   ,  \"τ1\" -> 0.015490030186   ,  \"τS\" -> 0.006638290269   ,  \"τN\" -> 0.000000433283   ,  \"τC\" -> 0.001884122649   ,  \"κ0\" -> 0.000000055099   ,  \"mm1\" -> 0.000027619939   ,  \"mm2\" -> 0.008620619838   ,  \"mm3\" -> 0.015491025321   ,  \"T\" -> 5.700000000000   ,  \"B\" -> 6.000000000000   ,  \"θ\" -> 90.000000000000   ,  \"Reoff\" -> 0.000000000000   ,  \"Imoff\" -> 0.000000000000   ,  \"στ1\" -> 0.134458541237   ,  \"στS\" -> 0.000000694139   ,  \"στN\" -> 0.000002640501   ,  \"τ11 \" -> 0.000000000000   ,  \"τ12\" -> 0.000000000000   ,  \"τ22\" -> 0.000000000000   ,  \"τN1\" -> 0.000000000000   ,  \"τN2\" -> 0.000000000000   ,  \"σηlogτ1 \" -> 0.085447105740   ,  \"σηlogτS\" -> 0.000000087953   ,  \"σηlogτN\" -> 0.122534708662   ,  \"σlogτ1\" -> 8.680327902656   ,  \"σlogτS\" -> 0.000104565901   ,  \"σlogτN\" -> 6.094171441911   ,  \"σητ1\" -> 0.001323578247   ,  \"σητS \" -> 0.000000000584   ,  \"σητN\" -> 0.000000053092    |>   , \n\"IDS0654_220613_RAW_cal__sam_\" ->   <|    \"ζ\" -> 0.000000000000   ,  \"τ1\" -> 0.000000000000   ,  \"τS\" -> 0.000000000000   ,  \"τN\" -> 0.000000000000   ,  \"τC\" -> 0.000000000000   ,  \"κ0\" -> 0.000000000000   ,  \"mm1\" -> 0.000000000000   ,  \"mm2\" -> 0.000000000000   ,  \"mm3\" -> 0.000000000000   ,  \"T\" -> 5.700000000000   ,  \"B\" -> 6.000000000000   ,  \"θ\" -> 90.000000000000   ,  \"Reoff\" -> 0.000000000000   ,  \"Imoff\" -> 0.000000000000   ,  \"στ1\" -> 0.000000000000   ,  \"στS\" -> 0.000000000000   ,  \"στN\" -> 0.000000000000   ,  \"τ11 \" -> 0.000000000000   ,  \"τ12\" -> 0.000000000000   ,  \"τ22\" -> 0.000000000000   ,  \"τN1\" -> 0.000000000000   ,  \"τN2\" -> 0.000000000000   ,  \"σηlogτ1 \" -> 0.000000000000   ,  \"σηlogτS\" -> 0.000000000000   ,  \"σηlogτN\" -> 0.000000000000   ,  \"σlogτ1\" -> 0.000000000000   ,  \"σlogτS\" -> 0.000000000000   ,  \"σlogτN\" -> 0.000000000000   ,  \"σητ1\" -> 0.000000000000   ,  \"σητS \" -> 0.000000000000   ,  \"σητN\" -> 0.000000000000    |>   , \n\"IDS0656_220614_RAW_cal__ref_\" ->   <|    \"ζ\" -> 0.110263031005   ,  \"τ1\" -> 0.036264946317   ,  \"τS\" -> 0.035363841561   ,  \"τN\" -> 0.002907549875   ,  \"τC\" -> 0.001147321567   ,  \"κ0\" -> 0.000000001565   ,  \"mm1\" -> 0.000111012610   ,  \"mm2\" -> 0.028483762528   ,  \"mm3\" -> 0.051308803802   ,  \"T\" -> 0.300000000000   ,  \"B\" -> 4.000000000000   ,  \"θ\" -> 90.000000000000   ,  \"Reoff\" -> 0.000000000000   ,  \"Imoff\" -> 0.000000000000   ,  \"στ1\" -> 0.000283051813   ,  \"στS\" -> 0.000006866298   ,  \"στN\" -> 0.000012798500   ,  \"τ11 \" -> 0.000000000000   ,  \"τ12\" -> 0.000000000000   ,  \"τ22\" -> 0.000000000000   ,  \"τN1\" -> 0.000000000000   ,  \"τN2\" -> 0.000000000000   ,  \"σηlogτ1 \" -> 0.116599052310   ,  \"σηlogτS\" -> 0.000355346389   ,  \"σηlogτN\" -> 0.130406494845   ,  \"σlogτ1\" -> 0.007805107735   ,  \"σlogτS\" -> 0.000194161553   ,  \"σlogτN\" -> 0.004401816116   ,  \"σητ1\" -> 0.004228458373   ,  \"σητS \" -> 0.000012566413   ,  \"σητN\" -> 0.000379163388    |>   , \n\"IDS0656_220614_RAW_cal__sam_\" ->   <|    \"ζ\" -> 0.000000000000   ,  \"τ1\" -> 0.000000000000   ,  \"τS\" -> 0.000000000000   ,  \"τN\" -> 0.000000000000   ,  \"τC\" -> 0.000000000000   ,  \"κ0\" -> 0.000000000000   ,  \"mm1\" -> 0.000000000000   ,  \"mm2\" -> 0.000000000000   ,  \"mm3\" -> 0.000000000000   ,  \"T\" -> 0.300000000000   ,  \"B\" -> 4.000000000000   ,  \"θ\" -> 90.000000000000   ,  \"Reoff\" -> 0.000000000000   ,  \"Imoff\" -> 0.000000000000   ,  \"στ1\" -> 0.000000000000   ,  \"στS\" -> 0.000000000000   ,  \"στN\" -> 0.000000000000   ,  \"τ11 \" -> 0.000000000000   ,  \"τ12\" -> 0.000000000000   ,  \"τ22\" -> 0.000000000000   ,  \"τN1\" -> 0.000000000000   ,  \"τN2\" -> 0.000000000000   ,  \"σηlogτ1 \" -> 0.000000000000   ,  \"σηlogτS\" -> 0.000000000000   ,  \"σηlogτN\" -> 0.000000000000   ,  \"σlogτ1\" -> 0.000000000000   ,  \"σlogτS\" -> 0.000000000000   ,  \"σlogτN\" -> 0.000000000000   ,  \"σητ1\" -> 0.000000000000   ,  \"σητS \" -> 0.000000000000   ,  \"σητN\" -> 0.000000000000    |>   , \n"
  in  "cspan":dbl=0.0001 format="%#_13g"
  in  "tab 13":enum32{"Page 1"}(tab)
  in  "alpha":dbl(slide)=0.19114213360578525 caption="ω0 (rad/sec)" scale=0.1..3.0 scale format="%#_2p"
  in  "apply RC transform":bool
  in  "tau":dbl(slide)=2.3809166168356322e-05 caption="ω0 (rad/sec)" scale=1e-08..0.01 scale format="%#_2p"
  in  "landscape plots":enum32{"Page 1", "Page 2"}(tab)
  in  "range one":dbl(slide)=0.006965 min=0.0 max=0.3 step=1e-06 scale=0.0001..1.0 scale format="%#_3p"
  in  "one":T1=enum."τS"
  out "Plot: goodness":cluster{"Freq out (Hz)":dbl[], dbl[]}[](graph)
  in  "plot landscape!":bool
  in  "range two":dbl(slide)=0.0039049999999999996 min=0.0 max=0.3 step=1e-06 scale=0.0001..1.0 scale format="%#_3p"
  in  "two":T1=enum."τ1"
  in  "what":enum16{"1d plots", "2d plots "}(ring)
  in  "# points":i32=200
  in  "Array":T1[](array[typedef])=[enum."ζ", enum."τ1", enum."τS", enum."τN", enum."τC"]
  in  "color Map":map{T1, u32}(c390)={enum."ζ"=7087058, enum."τ1"=56538, enum."τS"=2062078, enum."τN"=16740827, enum."τC"=16755712, enum."κ0"=11121611}
